vi "Write Class Data to File.vi"(8 "error in":errorcluster, 10 "filter":u8, 11 "CRDS Data in":refnum<class "CRDS Data.lvclass">) -> (0 "error out":errorcluster, 2 "binFileOut":refnum<file>, 3 "CRDS Data out":refnum<class "CRDS Data.lvclass">)   [LabVIEW 2014, in "CRDS Data.lvclass"]
uses:
  CRDS Data.lvclass
  CRDS Data.lvclass/CRDS Data.ctl
  crd_data_enum.ctl
  Cell/CRDS Cell Data.lvclass/CRDS Cell Data.ctl
  Data/Read measTime.vi
  Cell/CRDS Cell Data.lvclass
  File IO/File Utilities.lvlib
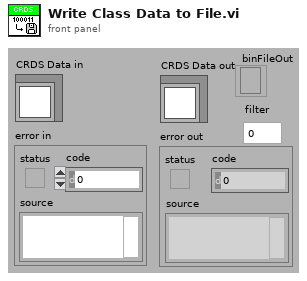
[diagram p1: front panel]
types:
  T1 = typedef "crd_data_enum.ctl" = enum8{"Time", "RHw", "TRH", "P", "Tmean", "RHsense", "TQ", "PQ", "Q", "Q0", "Qcal", "Qset", "extDilFac", "taucorr", "tau0corr", "stdevtau", "ext", "extCorr", "etau", "tau", "tau0", "Purge_Data", "NoData", "reserved", "Ttec", "Ang Exp", "Gamma", "filter", "fOverride", "notes", "max amp", "Tthermistor", "RhdilFac", "Psense", "TRHsense_bank", "RHsense_bank", "MFC_Data", "Thum", "ThumSP", "O3 Flow", "Pinlet Flow", "CLAP Flow", "O3 Add Valve", "O2 Valve", "O3 Cal"}
  T2 = enum16{"big-endian, network order", "native, host order", "little-endian"}
  T3 = typedef "calData.ctl" = cluster{"rhDilFac":sgl, "Q":sgl, "Tmean":sgl, "extDilFac":sgl, "rhCell":sgl, "P":sgl, "T":sgl}
  T4 = typedef "extparam.ctl" = cluster{"Tau":sgl, "Tau0cor":sgl, "ext":sgl, "extCorr":sgl, "stdevTau":sgl, "eTau":sgl, "taucorr":sgl, "Tau0":sgl, "max":sgl}
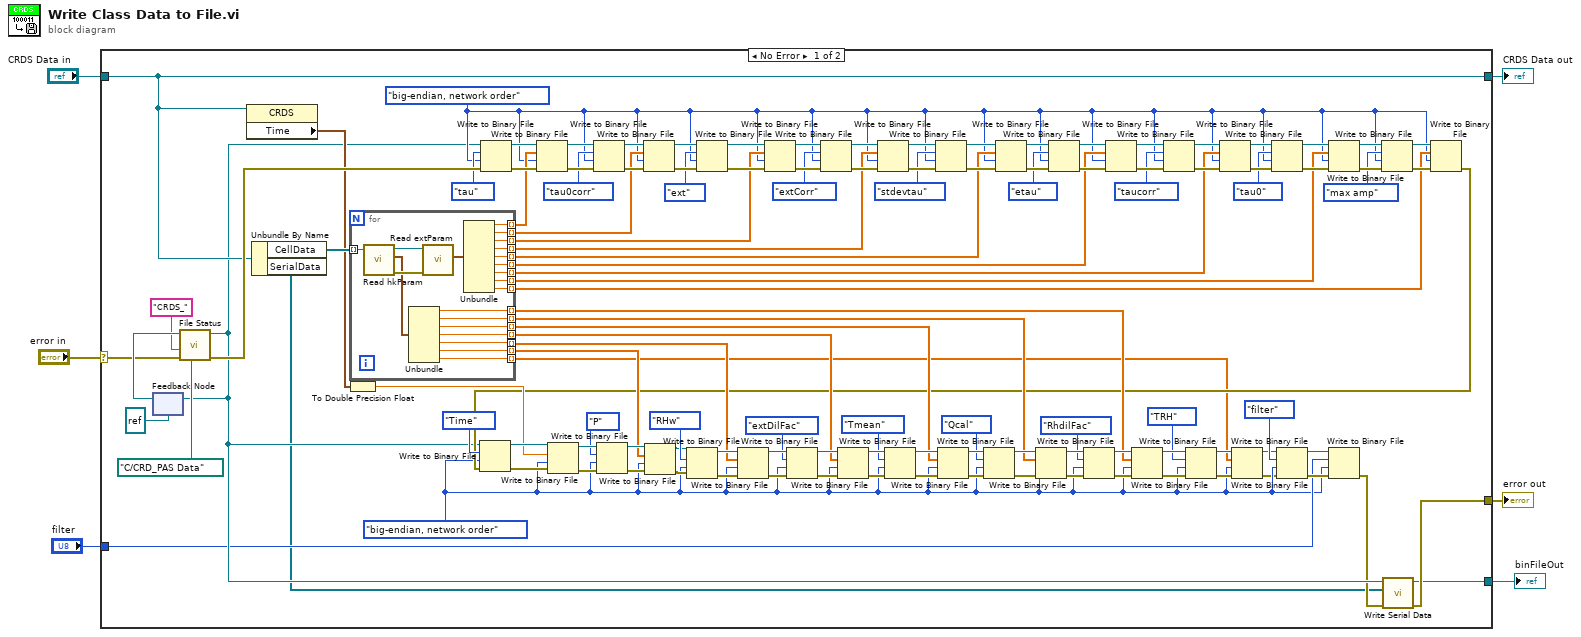
[diagram p0: block diagram]
diagram:
  n1 = case shown="No Error" "error in" {
    selector: "error in" -> [w122 w150]
    tunnel: [w127 w150] -> w5
    tunnel: [w22 w149] -> w3
    tunnel: "CRDS Data in" -> [w22 w149]
    tunnel: [w14 _] -> w2
    tunnel: "filter" -> [w12 _]
    frame No Error {
      w29 = T2."big-endian, network order" ("byte order (0:big-endian, network order)")
      w9 = T2."big-endian, network order" ("byte order (0:big-endian, network order)")
      n2 = feedback #1(refnum<file> refnum ("fileRefOut")) -> (w124:refnum<file>)
      n3 = call "File Status.vi"("Data Path"=path "C:/CRD_PAS Data", "erriorIn"=w122, "prefix"="CRDS_", "fileRefIn"=w124) -> ("error out"=w121:errorcluster, "fileRefOut"=w20:refnum<file>)  [unwired: 6 in]
      n4 = feedback-in #1(w20) -> ()
      n5 = property class="CRDS"(reference=w22) -> ("Time"=w21:timestamp)  [unwired: 1 in, 2 out]
      n6 = Unbundle By Name(w22) -> ("CellData"=w120:refnum<class "CRDS Cell Data.lvclass">[], "SerialData"=w10:refnum<class "Data.lvclass">[])
      n7 = To Double Precision Float(number=w21) -> (double precision float=w116:dbl)
      n8 = for {
        tunnel: w120 -> [w148] mode=indexing
        tunnel: [w144] -> w82 mode=indexing
        tunnel: [w143] -> w88 mode=indexing
        tunnel: [w142] -> w94 mode=indexing
        tunnel: [w141] -> w100 mode=indexing
        tunnel: [w140] -> w106 mode=indexing
        tunnel: [w139] -> w110 mode=indexing
        tunnel: [w137] -> w30 mode=indexing
        tunnel: [w136] -> w36 mode=indexing
        tunnel: [w135] -> w40 mode=indexing
        tunnel: [w134] -> w43 mode=indexing
        tunnel: [w133] -> w44 mode=indexing
        tunnel: [w132] -> w53 mode=indexing
        tunnel: [w131] -> w55 mode=indexing
        tunnel: [w130] -> w58 mode=indexing
        tunnel: [w129] -> w59 mode=indexing
        tunnel: [w128] -> w11 mode=indexing
        n9 = call "Read hkParam.vi"("CRDS Cell Data in"=w148) -> ("error out"=w146:errorcluster, "hkParam"=w145:T3, "CRDS Cell Data out"=w147:refnum<class "CRDS Cell Data.lvclass">)  [unwired: 8 in]
        n10 = Unbundle(w145) -> ("rhDilFac"=w144:sgl, "Q"=w143:sgl, "Tmean"=w142:sgl, "extDilFac"=w141:sgl, "rhCell"=w140:sgl, "P"=w139:sgl, "T"=w128:sgl)
        n11 = call "Read extParam.vi"("error in"=w146, "CRDS Cell Data in"=w147) -> ("extParam"=w138:T4)  [unwired: 7 in, 2 out]
        n12 = Unbundle(w138) -> ("Tau"=w129:sgl, "Tau0cor"=w130:sgl, "ext"=w131:sgl, "extCorr"=w132:sgl, "stdevTau"=w133:sgl, "eTau"=w134:sgl, "taucorr"=w135:sgl, "Tau0"=w136:sgl, "max"=w137:sgl)
      }
      n13 = Write to Binary File(file (use dialog)=w20, data=crd_data_enum."tau" ("CRD_Data_Enum"), error in=w121, 9:w29) -> (refnum out=w61:refnum<file>, error out=w63:errorcluster)  [unwired: 2 in, 1 out]
      n14 = Write to Binary File(file (use dialog)=w61, data=w59, error in=w63, 9:w29) -> (refnum out=w60:refnum<file>, error out=w64:errorcluster)  [unwired: 2 in, 1 out]
      n15 = Write to Binary File(file (use dialog)=w60, data=crd_data_enum."tau0corr" ("CRD_Data_Enum"), error in=w64, 9:w29) -> (refnum out=w57:refnum<file>, error out=w65:errorcluster)  [unwired: 2 in, 1 out]
      n16 = Write to Binary File(file (use dialog)=w57, data=w58, error in=w65, 9:w29) -> (refnum out=w56:refnum<file>, error out=w66:errorcluster)  [unwired: 2 in, 1 out]
      n17 = Write to Binary File(file (use dialog)=w56, data=crd_data_enum."ext" ("CRD_Data_Enum"), error in=w66, 9:w29) -> (refnum out=w54:refnum<file>, error out=w67:errorcluster)  [unwired: 2 in, 1 out]
      n18 = Write to Binary File(file (use dialog)=w54, data=w55, error in=w67, 9:w29) -> (refnum out=w51:refnum<file>, error out=w68:errorcluster)  [unwired: 2 in, 1 out]
      n19 = Write to Binary File(file (use dialog)=w51, data=crd_data_enum."extCorr" ("CRD_Data_Enum"), error in=w68, 9:w29) -> (refnum out=w52:refnum<file>, error out=w69:errorcluster)  [unwired: 2 in, 1 out]
      n20 = Write to Binary File(file (use dialog)=w52, data=w53, error in=w69, 9:w29) -> (refnum out=w50:refnum<file>, error out=w70:errorcluster)  [unwired: 2 in, 1 out]
      n21 = Write to Binary File(file (use dialog)=w50, data=crd_data_enum."stdevtau" ("CRD_Data_Enum"), error in=w70, 9:w29) -> (refnum out=w49:refnum<file>, error out=w71:errorcluster)  [unwired: 2 in, 1 out]
      n22 = Write to Binary File(file (use dialog)=w49, data=w44, error in=w71, 9:w29) -> (refnum out=w72:refnum<file>, error out=w73:errorcluster)  [unwired: 2 in, 1 out]
      n23 = Write to Binary File(file (use dialog)=w72, data=crd_data_enum."etau" ("CRD_Data_Enum"), error in=w73, 9:w29) -> (refnum out=w74:refnum<file>, error out=w75:errorcluster)  [unwired: 2 in, 1 out]
      n24 = Write to Binary File(file (use dialog)=w74, data=w43, error in=w75, 9:w29) -> (refnum out=w76:refnum<file>, error out=w77:errorcluster)  [unwired: 2 in, 1 out]
      n25 = Write to Binary File(file (use dialog)=w76, data=crd_data_enum."taucorr" ("CRD_Data_Enum"), error in=w77, 9:w29) -> (refnum out=w79:refnum<file>, error out=w78:errorcluster)  [unwired: 2 in, 1 out]
      n26 = Write to Binary File(file (use dialog)=w79, data=w40, error in=w78, 9:w29) -> (refnum out=w80:refnum<file>, error out=w81:errorcluster)  [unwired: 2 in, 1 out]
      n27 = Write to Binary File(file (use dialog)=w80, data=crd_data_enum."tau0" ("CRD_Data_Enum"), error in=w81, 9:w29) -> (refnum out=w38:refnum<file>, error out=w37:errorcluster)  [unwired: 2 in, 1 out]
      n28 = Write to Binary File(file (use dialog)=w38, data=w36, error in=w37, 9:w29) -> (refnum out=w35:refnum<file>, error out=w34:errorcluster)  [unwired: 2 in, 1 out]
      n29 = Write to Binary File(file (use dialog)=w35, data=crd_data_enum."max amp" ("CRD_Data_Enum"), error in=w34, 9:w29) -> (refnum out=w32:refnum<file>, error out=w31:errorcluster)  [unwired: 2 in, 1 out]
      n30 = Write to Binary File(file (use dialog)=w32, data=w30, error in=w31, 9:w29) -> (error out=w23:errorcluster)  [unwired: 2 in, 2 out]
      n31 = Write to Binary File(file (use dialog)=w20, data=crd_data_enum."Time" ("CRD_Data_Enum"), error in=w23, 9:w9) -> (refnum out=w117:refnum<file>, error out=w118:errorcluster)  [unwired: 2 in, 1 out]
      n32 = Write to Binary File(file (use dialog)=w117, data=w116, error in=w118, 9:w9) -> (refnum out=w115:refnum<file>, error out=w114:errorcluster)  [unwired: 2 in, 1 out]
      n33 = Write to Binary File(file (use dialog)=w115, data=crd_data_enum."P" ("CRD_Data_Enum"), error in=w114, 9:w9) -> (refnum out=w113:refnum<file>, error out=w112:errorcluster)  [unwired: 2 in, 1 out]
      n34 = Write to Binary File(file (use dialog)=w113, data=w110, error in=w112, 9:w9) -> (refnum out=w25:refnum<file>, error out=w24:errorcluster)  [unwired: 2 in, 1 out]
      n35 = Write to Binary File(file (use dialog)=w25, data=crd_data_enum."RHw" ("CRD_Data_Enum"), error in=w24, 9:w9) -> (refnum out=w108:refnum<file>, error out=w107:errorcluster)  [unwired: 2 in, 1 out]
      n36 = Write to Binary File(file (use dialog)=w108, data=w106, error in=w107, 9:w9) -> (refnum out=w105:refnum<file>, error out=w104:errorcluster)  [unwired: 2 in, 1 out]
      n37 = Write to Binary File(file (use dialog)=w105, data=crd_data_enum."extDilFac" ("CRD_Data_Enum"), error in=w104, 9:w9) -> (refnum out=w101:refnum<file>, error out=w102:errorcluster)  [unwired: 2 in, 1 out]
      n38 = Write to Binary File(file (use dialog)=w101, data=w100, error in=w102, 9:w9) -> (refnum out=w99:refnum<file>, error out=w98:errorcluster)  [unwired: 2 in, 1 out]
      n39 = Write to Binary File(file (use dialog)=w99, data=crd_data_enum."Tmean" ("CRD_Data_Enum"), error in=w98, 9:w9) -> (refnum out=w96:refnum<file>, error out=w95:errorcluster)  [unwired: 2 in, 1 out]
      n40 = Write to Binary File(file (use dialog)=w96, data=w94, error in=w95, 9:w9) -> (refnum out=w93:refnum<file>, error out=w92:errorcluster)  [unwired: 2 in, 1 out]
      n41 = Write to Binary File(file (use dialog)=w93, data=crd_data_enum."Qcal" ("CRD_Data_Enum"), error in=w92, 9:w9) -> (refnum out=w90:refnum<file>, error out=w89:errorcluster)  [unwired: 2 in, 1 out]
      n42 = Write to Binary File(file (use dialog)=w90, data=w88, error in=w89, 9:w9) -> (refnum out=w86:refnum<file>, error out=w87:errorcluster)  [unwired: 2 in, 1 out]
      n43 = Write to Binary File(file (use dialog)=w86, data=crd_data_enum."RhdilFac" ("CRD_Data_Enum"), error in=w87, 9:w9) -> (refnum out=w84:refnum<file>, error out=w83:errorcluster)  [unwired: 2 in, 1 out]
      n44 = Write to Binary File(file (use dialog)=w84, data=w82, error in=w83, 9:w9) -> (refnum out=w18:refnum<file>, error out=w19:errorcluster)  [unwired: 2 in, 1 out]
      n45 = Write to Binary File(file (use dialog)=w18, data=crd_data_enum."TRH" ("CRD_Data_Enum"), error in=w19, 9:w9) -> (refnum out=w16:refnum<file>, error out=w15:errorcluster)  [unwired: 2 in, 1 out]
      n46 = Write to Binary File(file (use dialog)=w16, data=w11, error in=w15, 9:w9) -> (refnum out=w8:refnum<file>, error out=w7:errorcluster)  [unwired: 2 in, 1 out]
      n47 = Write to Binary File(file (use dialog)=w8, data=crd_data_enum."filter" ("CRD_Data_Enum"), error in=w7, 9:w9) -> (refnum out=w27:refnum<file>, error out=w26:errorcluster)  [unwired: 2 in, 1 out]
      n48 = Write to Binary File(file (use dialog)=w27, data=w12, error in=w26, 9:w9) -> (error out=w13:errorcluster)  [unwired: 2 in, 2 out]
      n49 = call "Write Serial Data.vi"("error in"=w13, "SerialData"=w10, "binFile"=w20) -> ("error out"=w127:errorcluster, "binFileOut"=w14:refnum<file>)  [unwired: 6 in]
    }
    frame Error {
    }
  }
  "error out" <- w5
  "CRDS Data out" <- w3
  "binFileOut" <- w2
